vi "ex1.vi"() -> ()   [LabVIEW 2019]
panel:
  out "nbre de mois 2":dbl
  out "nbre de jours":dbl
  out "nbre d heures":dbl
  out "nbre de minutes":dbl
  in  "nbre de secondes":dbl
  in  "nbre de minutes 4":dbl
  out "nbre de secondes 4":dbl
  in  "nbre d heures 3":dbl
  out "nbre de secondes 3":dbl
  out "nbre de secondes 2":dbl
  in  "nbre de jrs 2":dbl
  out "nbre de secondes":dbl
  in  "nbre de mois":dbl
  in  "b":dbl(knob) scale=0.0..10.0
  in  "a":dbl(knob) scale=0.0..10.0
  out "Boolean":bool
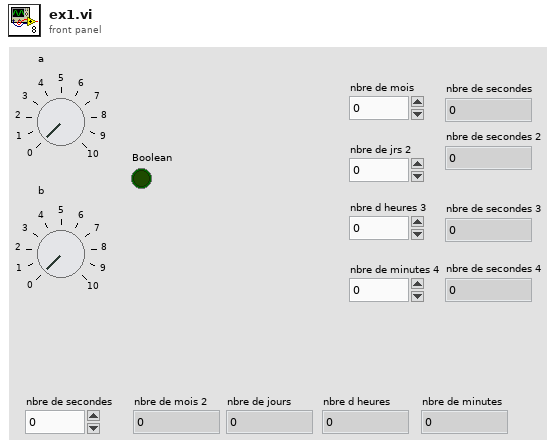
[diagram p1: front panel]
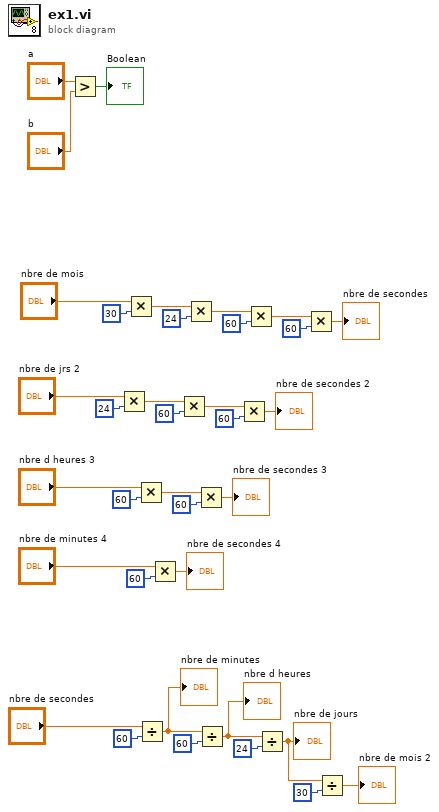
[diagram p0: block diagram]
diagram:
  n1 = Greater?(x="a", y="b") -> (0:→"Boolean":bool)
  n2 = Multiply(x="nbre de jrs 2", y=24) -> (x*y=w24:dbl)
  n3 = Multiply(x="nbre de mois", y=30) -> (x*y=w26:dbl)
  n4 = Multiply(x="nbre d heures 3", y=60) -> (x*y=w18:dbl)
  n5 = Divide(x="nbre de secondes", y=60) -> (x/y=w7:dbl)
  "nbre de minutes" <- w7
  n6 = Multiply(x="nbre de minutes 4", y=60) -> (x*y=→"nbre de secondes 4":dbl)
  n7 = Multiply(x=w24, y=60) -> (x*y=w10:dbl)
  n8 = Multiply(x=w26, y=24) -> (x*y=w30:dbl)
  n9 = Multiply(x=w18, y=60) -> (x*y=→"nbre de secondes 3":dbl)
  n10 = Divide(x=w7, y=60) -> (x/y=w4:dbl)
  "nbre d heures" <- w4
  n11 = Multiply(x=w10, y=60) -> (x*y=→"nbre de secondes 2":dbl)
  n12 = Multiply(x=w30, y=60) -> (x*y=w28:dbl)
  n13 = Divide(x=w4, y=24) -> (x/y=w2:dbl)
  "nbre de jours" <- w2
  n14 = Multiply(x=w28, y=60) -> (x*y=→"nbre de secondes":dbl)
  n15 = Divide(x=w2, y=30) -> (x/y=→"nbre de mois 2":dbl)
